vi "总磷总氮断电保存全局变量.vi"() -> ()   [LabVIEW 2016, in "斯坦道总磷总氮.lvlib"]
panel:
  in  "配置信息":T6 {"定点周期"."启动命令 24" items=["", "水样测试", "标样核查", "零点核查", "跨度核查", "空白测试", "平行样测试", "加标回收", "空白校准", "标样校准"]; "定点周期"."启动命令 23" items=["", "水样测试", "标样核查", "零点核查", "跨度核查", "空白测试", "平行样测试", "加标回收", "空白校准", "标样校准"]; "定点周期"."启动命令 22" items=["", "水样测试", "标样核查", "零点核查", "跨度核查", "空白测试", "平行样测试", "加标回收", "空白校准", "标样校准"]; "定点周期"."启动命令 21" items=["", "水样测试", "标样核查", "零点核查", "跨度核查", "空白测试", "平行样测试", "加标回收", "空白校准", "标样校准"]; "定点周期"."启动命令 20" items=["", "水样测试", "标样核查", "零点核查", "跨度核查", "空白测试", "平行样测试", "加标回收", "空白校准", "标样校准"]; "定点周期"."启动命令 19" items=["", "水样测试", "标样核查", "零点核查", "跨度核查", "空白测试", "平行样测试", "加标回收", "空白校准", "标样校准"]; "定点周期"."启动命令 18" items=["", "水样测试", "标样核查", "零点核查", "跨度核查", "空白测试", "平行样测试", "加标回收", "空白校准", "标样校准"]; "定点周期"."启动命令 17" items=["", "水样测试", "标样核查", "零点核查", "跨度核查", "空白测试", "平行样测试", "加标回收", "空白校准", "标样校准"]; "定点周期"."启动命令 16" items=["", "水样测试", "标样核查", "零点核查", "跨度核查", "空白测试", "平行样测试", "加标回收", "空白校准", "标样校准"]; "定点周期"."启动命令 15" items=["", "水样测试", "标样核查", "零点核查", "跨度核查", "空白测试", "平行样测试", "加标回收", "空白校准", "标样校准"]; "定点周期"."启动命令 14" items=["", "水样测试", "标样核查", "零点核查", "跨度核查", "空白测试", "平行样测试", "加标回收", "空白校准", "标样校准"]; "定点周期"."启动命令 13" items=["", "水样测试", "标样核查", "零点核查", "跨度核查", "空白测试", "平行样测试", "加标回收", "空白校准", "标样校准"]; "定点周期"."启动命令 12" items=["", "水样测试", "标样核查", "零点核查", "跨度核查", "空白测试", "平行样测试", "加标回收", "空白校准", "标样校准"]; "定点周期"."启动命令 11" items=["", "水样测试", "标样核查", "零点核查", "跨度核查", "空白测试", "平行样测试", "加标回收", "空白校准", "标样校准"]; "定点周期"."启动命令 10" items=["", "水样测试", "标样核查", "零点核查", "跨度核查", "空白测试", "平行样测试", "加标回收", "空白校准", "标样校准"]; "定点周期"."启动命令 9" items=["", "水样测试", "标样核查", "零点核查", "跨度核查", "空白测试", "平行样测试", "加标回收", "空白校准", "标样校准"]; "定点周期"."启动命令 8" items=["", "水样测试", "标样核查", "零点核查", "跨度核查", "空白测试", "平行样测试", "加标回收", "空白校准", "标样校准"]; "定点周期"."启动命令 7" items=["", "水样测试", "标样核查", "零点核查", "跨度核查", "空白测试", "平行样测试", "加标回收", "空白校准", "标样校准"]; "定点周期"."启动命令 6" items=["", "水样测试", "标样核查", "零点核查", "跨度核查", "空白测试", "平行样测试", "加标回收", "空白校准", "标样校准"]; "定点周期"."启动命令 5" items=["", "水样测试", "标样核查", "零点核查", "跨度核查", "空白测试", "平行样测试", "加标回收", "空白校准", "标样校准"]; "定点周期"."启动命令 4" items=["", "水样测试", "标样核查", "零点核查", "跨度核查", "空白测试", "平行样测试", "加标回收", "空白校准", "标样校准"]; "定点周期"."启动命令 3" items=["", "水样测试", "标样核查", "零点核查", "跨度核查", "空白测试", "平行样测试", "加标回收", "空白校准", "标样校准"]; "定点周期"."启动命令 2" items=["", "水样测试", "标样核查", "零点核查", "跨度核查", "空白测试", "平行样测试", "加标回收", "空白校准", "标样校准"]; "定点周期"."启动命令" items=["", "水样测试", "标样核查", "零点核查", "跨度核查", "空白测试", "平行样测试", "加标回收", "空白校准", "标样校准"]; "间隔启动"."启动命令" items=["", "水样测试", "标样核查", "零点核查", "跨度核查", "空白测试", "平行样测试", "加标回收", "空白校准", "标样校准"]}
  in  "总氮仪器参数":T7
  in  "总磷仪器参数":T7
  in  "MB通信方式选择":enum16{"串口", "TCP"}(ring)
  in  "PORT":string="1002"
  in  "IP":string="127.0.0.1"
  in  "VISA Resource":refnum<visa-resource-name>="COM5"
  in  "运行周期":T8={"运行模式"=enum."维护模式", "质控频次"=enum."关闭", "空白核查时间"=2, "跨度核查时间"=6, "24H周期设置"=[]} {"跨度核查时间" items=["00H", "01H", "02H", "03H", "04H", "05H", "06H", "07H", "08H", "09H", "10H", "11H", "12H", "13H", "14H", "15H", "16H", "17H", "18H", "19H", "20H", "21H", "22H", "23H", "关闭"]; "空白核查时间" items=["00H", "01H", "02H", "03H", "04H", "05H", "06H", "07H", "08H", "09H", "10H", "11H", "12H", "13H", "14H", "15H", "16H", "17H", "18H", "19H", "20H", "21H", "22H", "23H", "关闭"]}
  in  "流程路径":path=path "C:/Users/std/Documents/斯坦道流程文件/流程.xml"
  in  "总氮自动测试量程配置":T9={"水样测试量程模式"=enum."AUTO", "空白核查量程模式"=enum."AUTO", "跨度核查量程模式"=enum."AUTO"}
  in  "质控参数设置":T10
  in  "总磷自动测试量程配置":T9={"水样测试量程模式"=enum."AUTO", "空白核查量程模式"=enum."AUTO", "跨度核查量程模式"=enum."AUTO"}
  # "分钟"
  # "次"
  # "运行模式："
  # "质控频次："
  # "零点核查时间："
  # "跨度核查时间："
  # "质控参数设置"
  # "总氮"
  # "监测参数"
  # "总磷"
  # "跨度值"
  # "零点核查标准液浓度"
  # "跨度核查标准液浓度"
  # "标样核查标准液浓度"
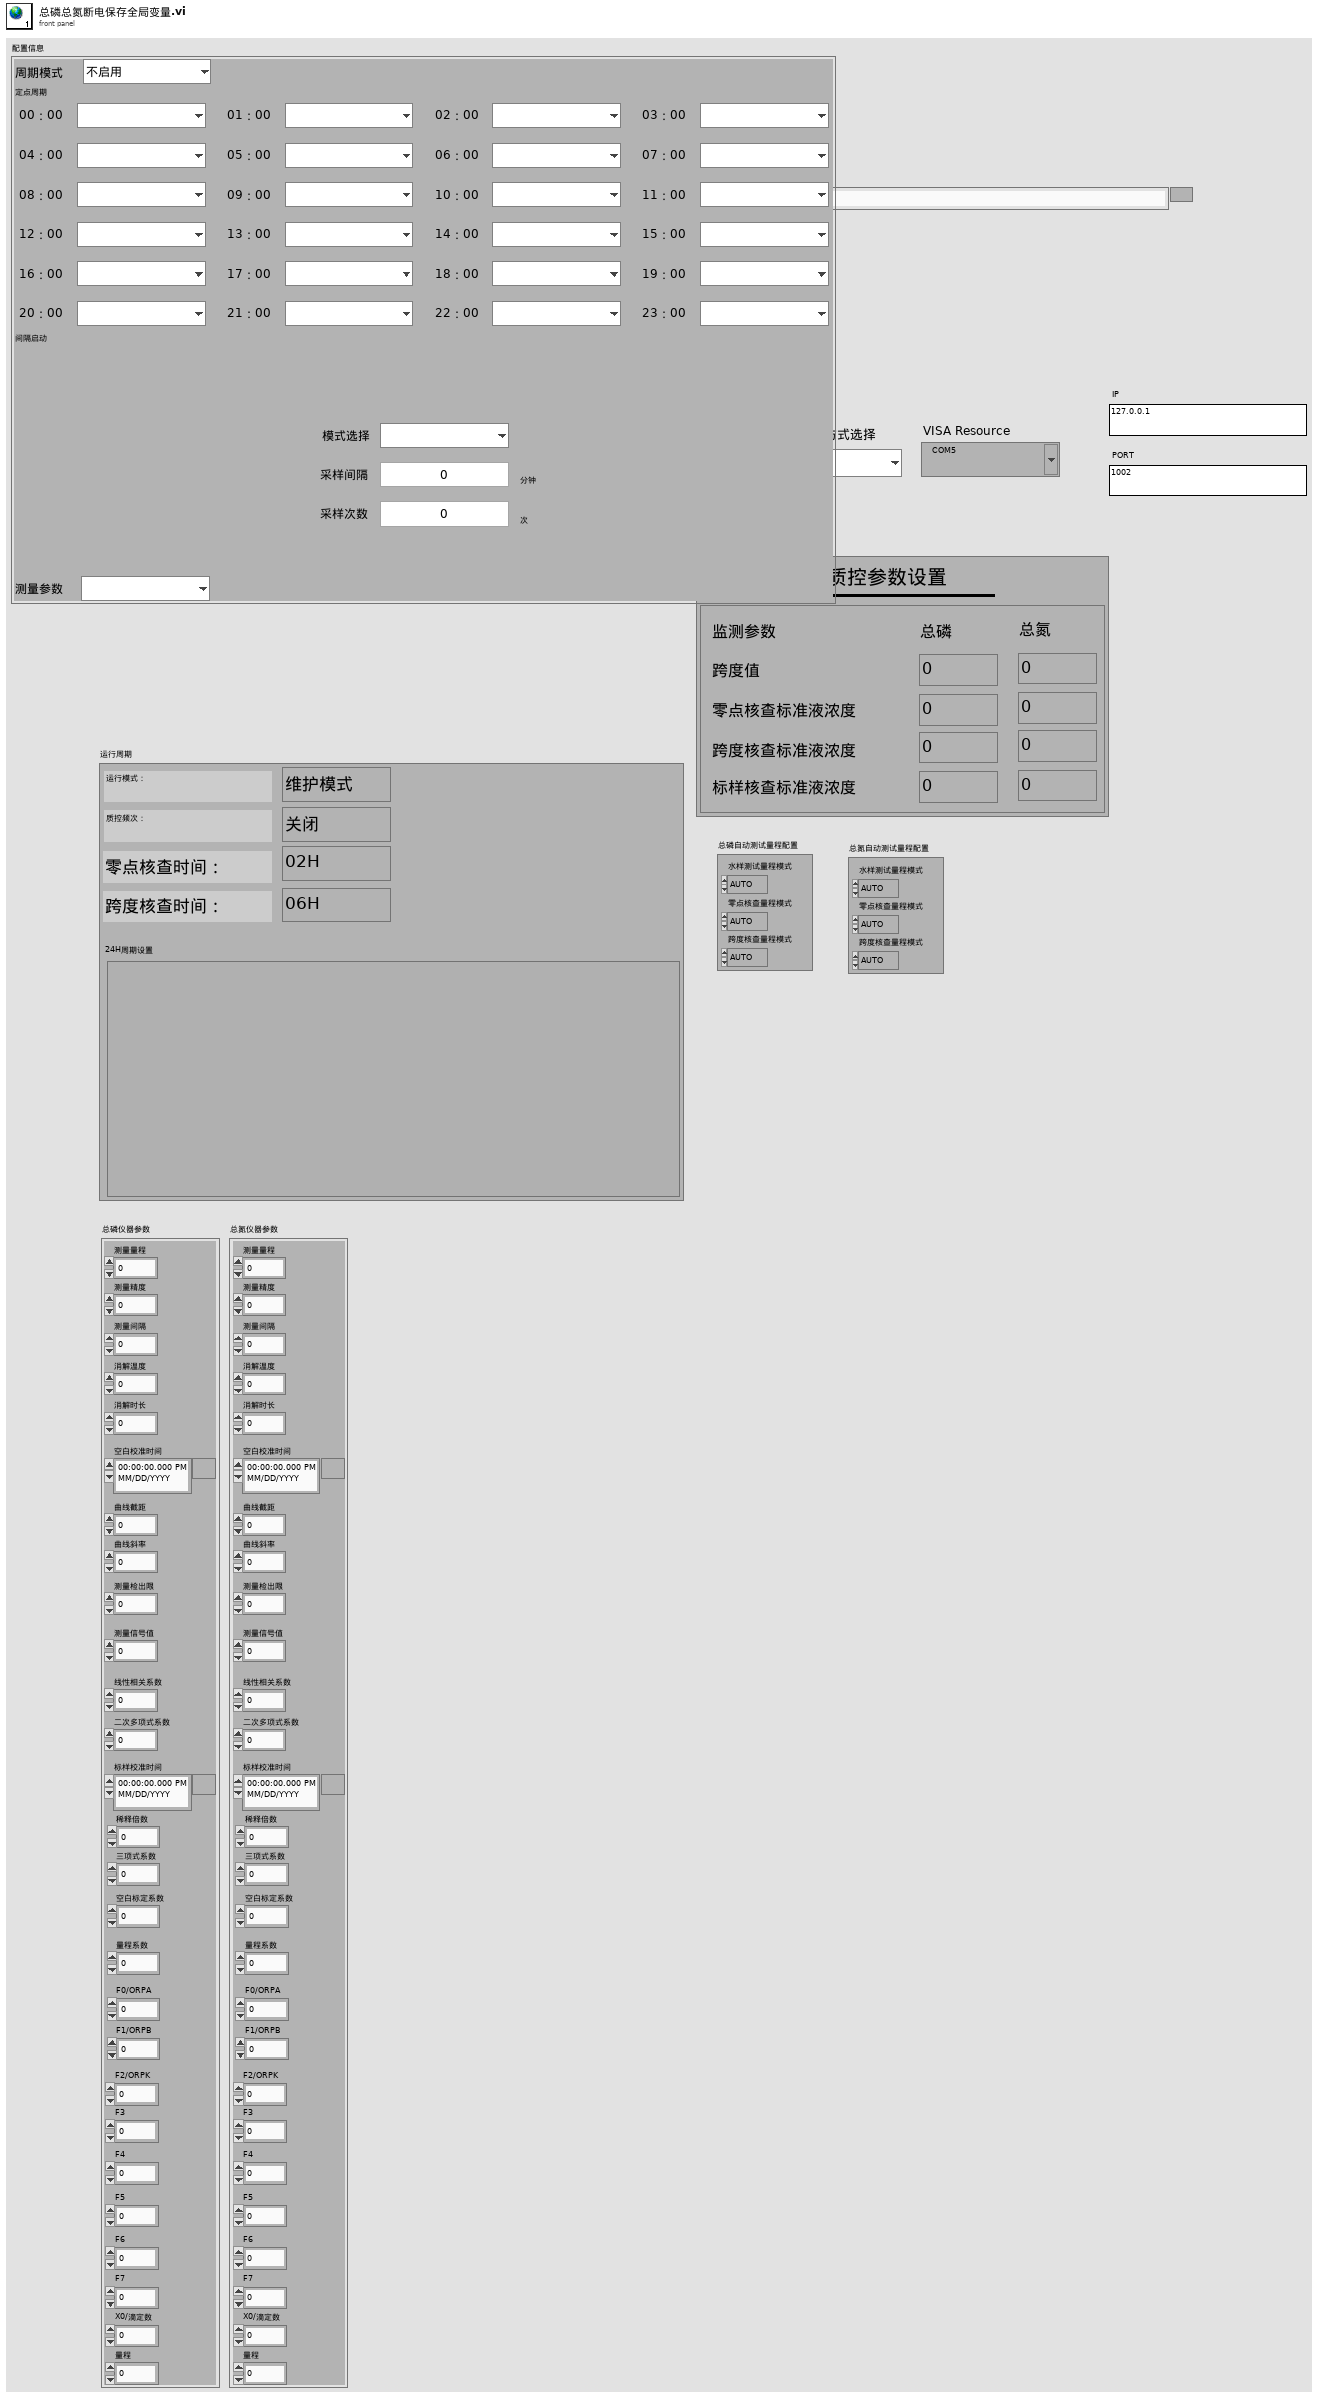
[diagram p1: front panel]
types:
  T1 = typedef "定时设置.xctl/周期模式设置.ctl" = enum16{"不启用", "定点模式", "间隔模式"}
  T2 = typedef "定时设置.xctl/定点周期设置.ctl" = cluster{"启动命令":T3, "启动命令 2":T3, "启动命令 3":T3, "启动命令 4":T3, "启动命令 5":T3, "启动命令 6":T3, "启动命令 7":T3, "启动命令 8":T3, "启动命令 9":T3, "启动命令 10":T3, "启动命令 11":T3, "启动命令 12":T3, "启动命令 13":T3, "启动命令 14":T3, "启动命令 15":T3, "启动命令 16":T3, "启动命令 17":T3, "启动命令 18":T3, "启动命令 19":T3, "启动命令 20":T3, "启动命令 21":T3, "启动命令 22":T3, "启动命令 23":T3, "启动命令 24":T3}
  T3 = typedef "定时设置.xctl/启动命令选择.ctl" = u16
  T4 = typedef "定时设置.xctl/间隔启动设置.ctl" = cluster{"启动命令":T3, "启动间隔":dbl, "启动次数":i32}
  T5 = typedef "定时设置.xctl/测量参数.ctl" = u16
  T6 = cluster{"周期模式":T1, "定点周期":T2, "间隔启动":T4, "测量参数":T5}
  T7 = cluster{"测量量程":dbl, "测量精度":dbl, "测量间隔":dbl, "消解温度":dbl, "消解时长":dbl, "空白校准时间":timestamp, "曲线截距":dbl, "曲线斜率":dbl, "测量检出限":dbl, "测量信号值":dbl, "线性相关系数":dbl, "二次多项式系数":dbl, "标样校准时间":timestamp, "稀释倍数":dbl, "三项式系数":dbl, "空白标定系数":dbl, "量程系数":dbl, "F0/ORPA":dbl, "F1/ORPB":dbl, "F2/ORPK":dbl, "F3":dbl, "F4":dbl, "F5":dbl, "F6":dbl, "F7":dbl, "X0/滴定数":dbl, "量程":dbl}
  T8 = cluster{"运行模式":enum16{"维护模式", "常规模式", "应急模式", "质控模式"}, "质控频次":enum16{"关闭", "每天", "星期一", "星期二", "星期三", "星期四", "星期五", "星期六", "星期日"}, "空白核查时间":u16, "跨度核查时间":u16, "24H周期设置":bool[]}
  T9 = cluster{"水样测试量程模式":enum16{"H", "L", "AUTO"}, "空白核查量程模式":enum16{"H", "L", "AUTO"}, "跨度核查量程模式":enum16{"H", "L", "AUTO"}}
  T10 = cluster{"总磷跨度值":dbl, "总磷零点标准液浓度":dbl, "总磷跨度标准液浓度":dbl, "总磷标准液标准浓度":dbl, "总氮跨度值":dbl, "总氮零点标准液浓度":dbl, "总氮跨度标准液浓度":dbl, "总氮标准液标准浓度":dbl}
diagram:
